vi "v0.2_lee_enc_http.vi"(8 "error in":errorcluster, 11 "mbed.lvclass IN":refnum<class "mbed.lvclass">) -> (0 "error out":errorcluster, 2 "angulo":i32, 3 "mbed.lvclass OUT":refnum<class "mbed.lvclass">)   [LabVIEW 2011]
doc: "<B>Servo ON</B>\n\nEncender/Apagar el servomotor utilizando una variable boolena"
uses:
  C:/mbed/Transport Mechanisms/mbed/mbed.lvclass
  C:/mbed/mbed Interface/RPCFunction/RPCFunction.lvclass
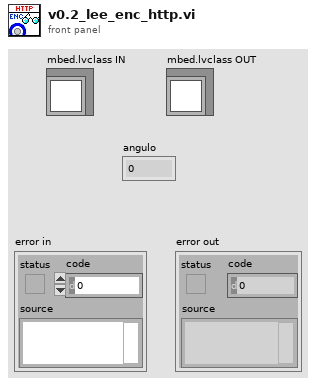
[diagram p1: front panel]
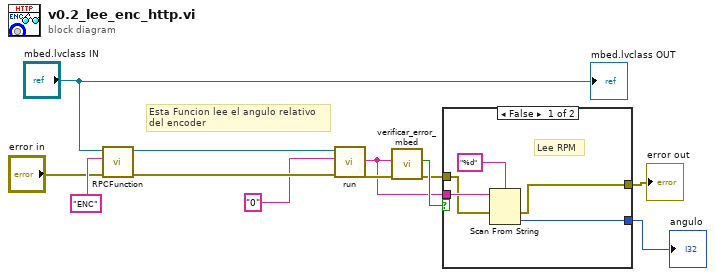
[diagram p0: block diagram]
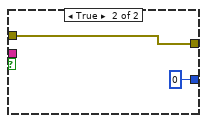
[diagram p2: hidden frame]
diagram:
  # "Esta Funcion lee el angulo relativo \ndel encoder"
  n1 = call "RPCFunction.vi"("error in (no error)"="error in", "Existing Obj Name"="ENC", "mbed_LVLibrary.lvlib:mbed.lvclass"="mbed.lvclass IN") -> ("error out"=w7:errorcluster, "mbed_LVLibrary.lvlib:Packet.lvclass 2"=w11:refnum<class "RPCFunction.lvclass">)  [unwired: 6 in, 1 out]
  n2 = call "run.vi"("error in (no error)"=w7, "Input"="0", "Packet in"=w11) -> ("error out"=w9:errorcluster, "Output"=w4:string)  [unwired: 6 in, 1 out]
  n3 = call "verificar_error_mbed.vi"("error in (no error)"=w9, "desde_mbed"=w4) -> ("error out"=w2:errorcluster, "error?"=w5:bool)  [unwired: 8 in]
  n4 = case shown="False" w5 {
    tunnel: w4 -> [w17 _]
    tunnel: [w14 w19] -> w3
    tunnel: w2 -> [w15 w19]
    tunnel: [w13 0] -> w1
    frame False {
      # "Lee RPM"
      n5 = Scan From String(format string="%d", input string=w17, error in=w15) -> (error out=w14:errorcluster, output 1=w13:i32)  [unwired: 2 in, 2 out]
    }
    frame True {
    }
  }
  "error out" <- w3
  "angulo" <- w1
  "mbed.lvclass OUT" <- "mbed.lvclass IN"
